vi "TestVirtual6.vi"(0 "reference in":refnum<class "G#SubClass1.lvclass">, 5 "error in (no error)":errorcluster) -> (14 "reference out":refnum<class "G#SubClass1.lvclass">, 15 "MethodName":string[](array[string]), 19 "error out":errorcluster)   [LabVIEW 2017, in "G#SubClass1.lvclass"]
uses:
  G#SubClass1.lvclass
  G#BaseClass1_class/G#BaseClass1.lvclass
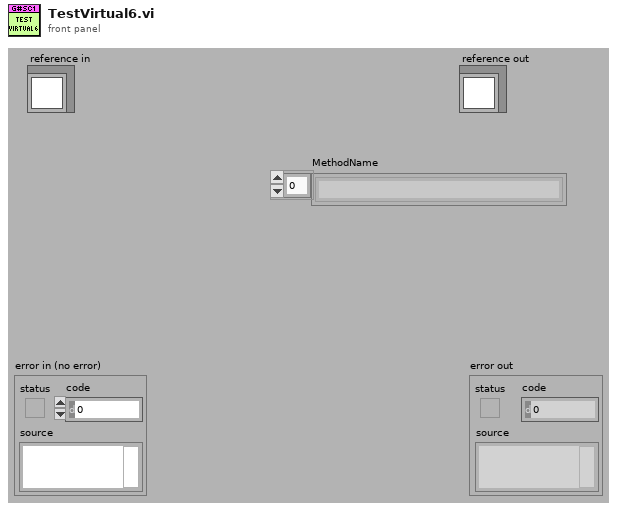
[diagram p1: front panel]
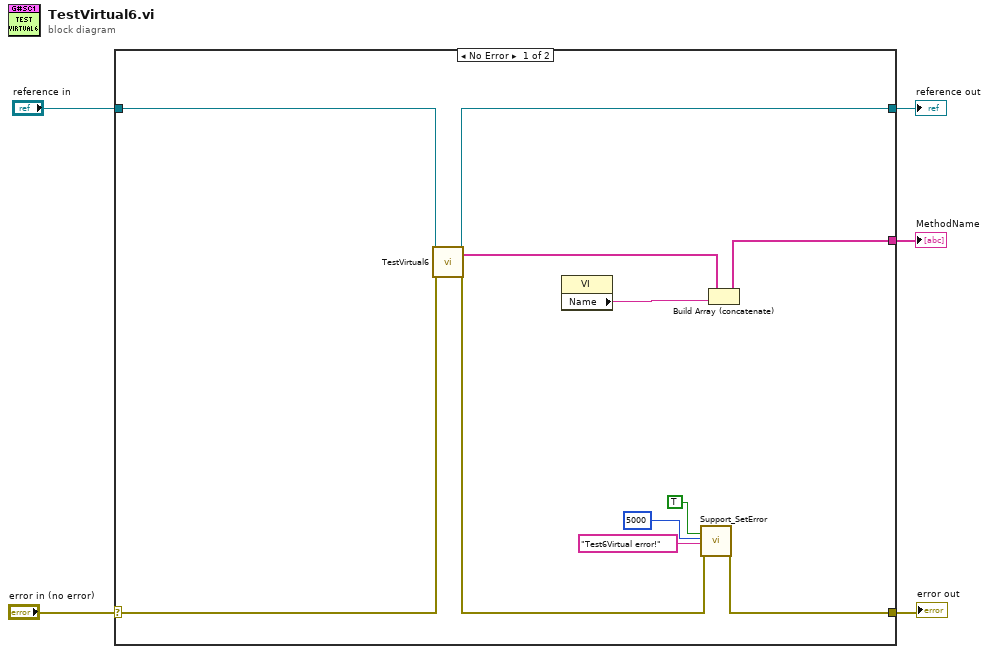
[diagram p0: block diagram]
diagram:
  n1 = case shown="No Error" "error in (no error)" {
    selector: "error in (no error)" -> [w16 w18]
    tunnel: [w6 w18] -> w4
    tunnel: [w14 w17] -> w2
    tunnel: "reference in" -> [w15 w17]
    tunnel: [w11 _] -> w1
    frame No Error {
      n2 = call-parent "TestVirtual6.vi"("reference in"=w15, "error in (no error)"=w16) -> ("reference out"=w14:refnum<class "G#SubClass1.lvclass">, "MethodName"=w12:string[], "error out"=w7:errorcluster)  [unwired: 15 in]
      n3 = property class="VI"() -> ("Name"=w13:string)  [unwired: 2 in, 2 out]
      n4 = call "Support_SetError.vi"("status"=TRUE, "code (5000)"=5000, "source"="Test6Virtual error!", "error in (no error)"=w7) -> ("error out"=w6:errorcluster)  [unwired: 15 in]
      n5 = Build Array (concatenate)(w12, w13) -> (w11:string[])
    }
    frame Error {
    }
  }
  "error out" <- w4
  "reference out" <- w2
  "MethodName" <- w1
